vi "Contours.vi"() -> ()   [LabVIEW 2018]
doc: "Contours: This example is an example of object contour recognition. In image processing and computer vision, contours refer to continuous boundary lines in an image that identify the shape and boundaries of an object or region. A contour is usually composed of a series of adjacent pixels or curves, which can be represented as closed or open curves. Contour plays an important role in image processing and can be used for various tasks such as object detection, segmentation, recognition, etc. By detecting the contours in an image, object shape information can be extracted, enabling operations such as object localization, counting, and classification."
uses:
  vi.lib/VIRobotics/opencv_yiku/ctls/ColorConversionCodes.ctl
  vi.lib/VIRobotics/opencv_yiku/Mat/Mat_8U/Mat_8U.lvclass
  D:/Program Files/Company/National Instruments/LabVIEW 2018(64bit)/vi.lib/addons/VIRobotics/opencv_yiku/Mat/Mat/Mat.lvclass
  vi.lib/VIRobotics/opencv_yiku/Mat/Create_Mat_8U.vi
  vi.lib/VIRobotics/opencv_yiku/opencv_yiku.lvlib
panel:
  out "带轮廓的图":picture
  out "二值化图":picture
  out "picture":picture
  # "Overview: Demonstrates how to find and draw Contours\nRequirements: Windows.\nInstructions: \n1.Run the VI"
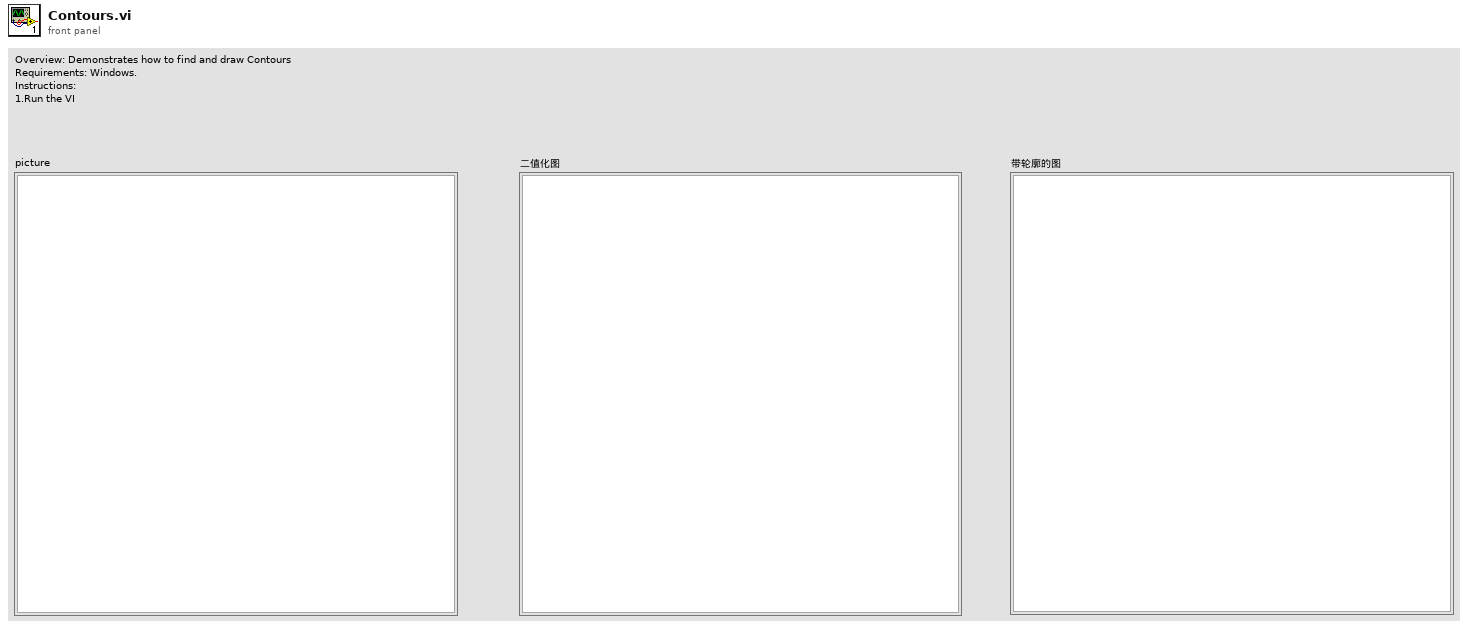
[diagram p1: front panel]
types:
  T1 = typedef "opencv_yiku.lvlib/ColorConversionCodes.ctl" = enum32{"COLOR_BGR2BGRA", "COLOR_BGRA2BGR", "COLOR_BGR2RGBA", "COLOR_RGBA2BGR", "COLOR_BGR2RGB", "COLOR_BGRA2RGBA", "COLOR_BGR2GRAY", "COLOR_RGB2GRAY", "COLOR_GRAY2BGR", "COLOR_GRAY2BGRA", "COLOR_BGRA2GRAY", "COLOR_RGBA2GRAY", "COLOR_BGR2BGR565", "COLOR_RGB2BGR565", "COLOR_BGR5652BGR", "COLOR_BGR5652RGB", "COLOR_BGRA2BGR565", "COLOR_RGBA2BGR565", "COLOR_BGR5652BGRA", "COLOR_BGR5652RGBA", "COLOR_GRAY2BGR565", "COLOR_BGR5652GRAY", "COLOR_BGR2BGR555", "COLOR_RGB2BGR555", "COLOR_BGR5552BGR", "COLOR_BGR5552RGB", "COLOR_BGRA2BGR555", "COLOR_RGBA2BGR555", "COLOR_BGR5552BGRA", "COLOR_BGR5552RGBA", "COLOR_GRAY2BGR555", "COLOR_BGR5552GRAY", "COLOR_BGR2XYZ", "COLOR_RGB2XYZ", "COLOR_XYZ2BGR", "COLOR_XYZ2RGB", "COLOR_BGR2YCrCb", "COLOR_RGB2YCrCb", "COLOR_YCrCb2BGR", "COLOR_YCrCb2RGB", "COLOR_BGR2HSV", "COLOR_RGB2HSV", "42", "43", "COLOR_BGR2Lab", "COLOR_RGB2Lab"}
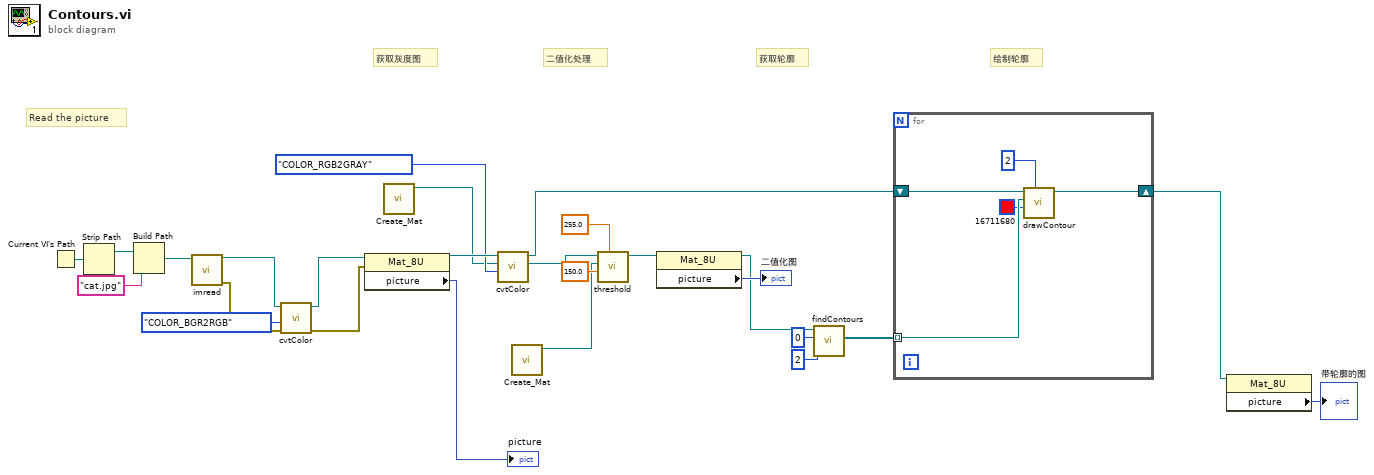
[diagram p0: block diagram]
diagram:
  # "Read the picture"
  # "绘制轮廓"
  # "获取轮廓"
  # "二值化处理"
  # "获取灰度图"
  n1 = Current VI's Path() -> (path=w24:path)
  n2 = Strip Path(path=w24) -> (stripped path=w26:path)  [unwired: 1 out]
  n3 = Build Path(base path=w26, name or relative path="cat.jpg") -> (appended path=w23:path)
  n4 = call "imread.vi"("path"=w23) -> ("error out"=w3:errorcluster, "Mat out"=w5:refnum<class "Mat_8U.lvclass">)  [unwired: 9 in]
  n5 = call "cvtColor.vi"("error in (no error)"=w3, "dstCn"=ColorConversionCodes."COLOR_BGR2RGB", "src"=w5) -> ("error out"=w2:errorcluster, "src out"=w4:refnum<class "Mat_8U.lvclass">)  [unwired: 6 in, 1 out]
  n6 = property class="Mat_8U"(reference=w4, error in=w2) -> (reference out=w21:refnum<class "Mat_8U.lvclass">, "picture"=→"picture":picture)  [unwired: 1 out]
  n7 = call-poly "Create_Mat.vi"() -> ("Mat_8U_out"=w10:refnum<class "Mat_8U.lvclass">)  [unwired: 10 in, 1 out]
  n8 = call "cvtColor.vi"("dstCn"=ColorConversionCodes."COLOR_RGB2GRAY", "dst"=w10, "src"=w21) -> ("dst out"=w9:refnum<class "Mat_8U.lvclass">, "src out"=w8:refnum<class "Mat_8U.lvclass">)  [unwired: 6 in, 1 out]
  n9 = call-poly "Create_Mat.vi"() -> ("Mat_8U_out"=w17:refnum<class "Mat_8U.lvclass">)  [unwired: 10 in, 1 out]
  n10 = call "threshold.vi"("maxval"=255.0, "thresh"=150.0, "dst in"=w17, "Mat in"=w9) -> ("dst out"=w16:refnum<class "Mat_8U.lvclass">)  [unwired: 6 in, 1 out]
  n11 = property class="Mat_8U"(reference=w16) -> (reference out=w14:refnum<class "Mat_8U.lvclass">, "picture"=→"二值化图":picture)  [unwired: 1 in, 1 out]
  n12 = call "findContours.vi"("method"=2, "mode"=0, "Mat in"=w14) -> ("Array"=w11:refnum<class "vector_Point.lvclass">[])  [unwired: 6 in, 2 out]
  n13 = for {
    tunnel: w11 -> [w31] mode=indexing
    shift-right: [w29] -> w7
    shift-left: w8 -> [w30]
    n14 = call "drawContour.vi"("thickness"=2, "Color"=u32 16711680, "vector<Point> in"=w31, "Mat in"=w30) -> ("Mat out"=w29:refnum<class "Mat_8U.lvclass">)  [unwired: 6 in, 1 out]
  }
  n15 = property class="Mat_8U"(reference=w7) -> ("picture"=→"带轮廓的图":picture)  [unwired: 1 in, 2 out]
